vi "Muscolino_v1_KCL.vi"() -> ()   [LabVIEW 2011]
uses:
  <vilib>/DAQmx/read.llb/DAQmx Read (Analog 1D Wfm NChan NSamp).vi
  <vilib>/DAQmx/create/channels.llb/DAQmx Create Channel (AI-Voltage-Basic).vi
  <vilib>/DAQmx/configure/timing.llb/DAQmx Timing (Sample Clock).vi
  <vilib>/DAQmx/configure/task.llb/DAQmx Configure Logging (TDMS).vi
  <vilib>/DAQmx/miscellaneous.llb/DAQmx Fill In Error Info.vi
panel:
  in  "Stimulator":T1={"frequency (Hz)"=1.0, "initial delay (ms)"=100.0, "# Stimuli"=2, "ON-OFF"=TRUE, "pulse dur (ms)"=2.0} {"frequency (Hz)" min=1.0 max=200.0 step=1.0 scale=0.0..100.0}
  in  "Read streamed data":bool
  in  "Play Button":bool
  out "Boolean":bool
  in  "Stop Button":bool
  out "Detector":bool=TRUE
  out "Shutters":bool=TRUE
  in  "Tab Control 3":enum32{"Continuous", "Finite sampling"}(tab)
  in  "ms/point":dbl=1.0
  in  "file path":path=path "C:/Users/Luca/Desktop/BABY"
  in  "ms/point 2":dbl=0.1
  in  "duration (ms)":i32=3000
  in  "Tab Control 2":enum32{"Shutters", "Detector TRG"}(tab)
  in  "Shutter #1":T2={"Duration (ms)"=770.0, "Delay (ms)"=910.0, "# Cycles"=1, "period (ms)"=500.0, "ENABLE"=FALSE}
  in  "Shutter #2":T2={"Duration (ms)"=3.0, "Delay (ms)"=918.0, "# Cycles"=1, "period (ms)"=500.0, "ENABLE"=FALSE}
  in  "TRG detector":T3={"Delay (ms)"=900.0, "Duration (ms)"=1.0, "ENABLE"=TRUE}
  in  "Tab Control":T4(tab)
  out "Waveform Chart 2":waveform(dbl)[](graph)=[{"t0"=timestamp(3645626346.405727 s since 1904-01-01), "dt"=0.001, "Y"=[-0.06398468896060096, -0.06242254708157085, -0.06554683084097776, -0.0664841159698506, -0.06773382947576925, -0.062110118705926365, -0.06273497545726918, -0.06429711733656855, -0.061797690330335706, -0.05929826332754758], "attributes"=variant("NI_ChannelName"=variant(string "Force"), "NI_UnitDescription"=variant(string "Volts"))}, {"t0"=timestamp(3645626346.405727 s since 1904-01-01), "dt"=0.001, "Y"=[10.23122258005124, 10.23122258005124, 10.23122258005124, 10.23122258005124, 10.23122258005124, 10.23122258005124, 10.23122258005124, 10.23122258005124, 10.23122258005124, 10.23122258005124], "attributes"=variant("NI_ChannelName"=variant(string "Motor"), "NI_UnitDescription"=variant(string "Volts"))}, {"t0"=timestamp(3645626346.405727 s since 1904-01-01), "dt"=0.001, "Y"=[0.001985937762198508, 0.01605118530383799, 0.02261496751857621, 0.028241066574480733, 0.03105411610756004, 0.028866188692646493, 0.03636765412387749, 0.02230240646031397, 0.022927528576880348, 0.009174842050874644], "attributes"=variant("NI_ChannelName"=variant(string "Stimulus"), "NI_UnitDescription"=variant(string "Volts"))}]
  out "Waveform Chart":waveform(dbl)[](graph)=[{"t0"=timestamp(3645626346.405727 s since 1904-01-01), "dt"=0.001, "Y"=[-0.06398468896060096, -0.06242254708157085, -0.06554683084097776, -0.0664841159698506, -0.06773382947576925, -0.062110118705926365, -0.06273497545726918, -0.06429711733656855, -0.061797690330335706, -0.05929826332754758], "attributes"=variant("NI_ChannelName"=variant(string "Force"), "NI_UnitDescription"=variant(string "Volts"))}, {"t0"=timestamp(3645626346.405727 s since 1904-01-01), "dt"=0.001, "Y"=[10.23122258005124, 10.23122258005124, 10.23122258005124, 10.23122258005124, 10.23122258005124, 10.23122258005124, 10.23122258005124, 10.23122258005124, 10.23122258005124, 10.23122258005124], "attributes"=variant("NI_ChannelName"=variant(string "Motor"), "NI_UnitDescription"=variant(string "Volts"))}, {"t0"=timestamp(3645626346.405727 s since 1904-01-01), "dt"=0.001, "Y"=[0.001985937762198508, 0.01605118530383799, 0.02261496751857621, 0.028241066574480733, 0.03105411610756004, 0.028866188692646493, 0.03636765412387749, 0.02230240646031397, 0.022927528576880348, 0.009174842050874644], "attributes"=variant("NI_ChannelName"=variant(string "Stimulus"), "NI_UnitDescription"=variant(string "Volts"))}]
  out "Waveform Graph":waveform(dbl)[](graph)=[{"t0"=timestamp(3645626338.6502304 s since 1904-01-01), "dt"=9.999999999999999e-05, "Y"=array[30000 elements], "attributes"=variant("NI_ChannelName"=variant(string "Force"), "NI_UnitDescription"=variant(string "Volts"))}, {"t0"=timestamp(3645626338.6502304 s since 1904-01-01), "dt"=9.999999999999999e-05, "Y"=array[30000 elements], "attributes"=variant("NI_ChannelName"=variant(string "Motor"), "NI_UnitDescription"=variant(string "Volts"))}, {"t0"=timestamp(3645626338.6502304 s since 1904-01-01), "dt"=9.999999999999999e-05, "Y"=array[30000 elements], "attributes"=variant("NI_ChannelName"=variant(string "Stimulus"), "NI_UnitDescription"=variant(string "Volts"))}, {"t0"=timestamp(3645626338.6502304 s since 1904-01-01), "dt"=9.999999999999999e-05, "Y"=array[30000 elements], "attributes"=variant("NI_ChannelName"=variant(string "SH1"), "NI_UnitDescription"=variant(string "Volts"))}, {"t0"=timestamp(3645626338.6502304 s since 1904-01-01), "dt"=9.999999999999999e-05, "Y"=array[30000 elements], "attributes"=variant("NI_ChannelName"=variant(string "SH2"), "NI_UnitDescription"=variant(string "Volts"))}, {"t0"=timestamp(3645626338.6502304 s since 1904-01-01), "dt"=9.999999999999999e-05, "Y"=array[30000 elements], "attributes"=variant("NI_ChannelName"=variant(string "TFG"), "NI_UnitDescription"=variant(string "Volts"))}, {"t0"=timestamp(3645626338.6502304 s since 1904-01-01), "dt"=9.999999999999999e-05, "Y"=array[30000 elements], "attributes"=variant("NI_ChannelName"=variant(string "PIN_DIODE"), "NI_UnitDescription"=variant(string "Volts"))}]
  # "STIMULATOR"
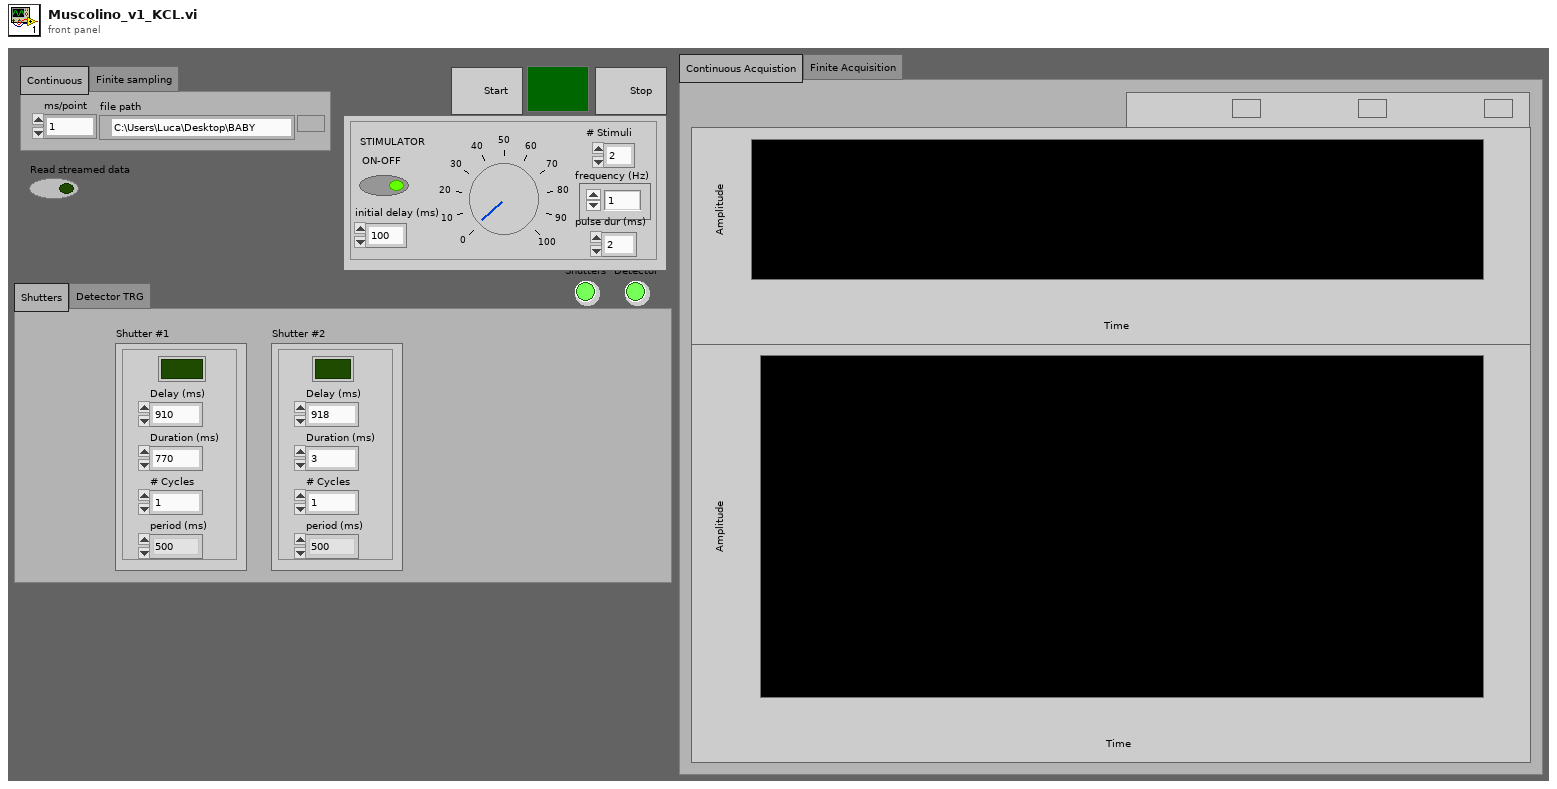
[diagram p1: front panel]
types:
  T1 = cluster{"frequency (Hz)":dbl, "initial delay (ms)":dbl, "# Stimuli":i8, "ON-OFF":bool, "pulse dur (ms)":dbl}
  T2 = cluster{"Duration (ms)":dbl, "Delay (ms)":dbl, "# Cycles":i8, "period (ms)":dbl, "ENABLE":bool}
  T3 = cluster{"Delay (ms)":dbl, "Duration (ms)":dbl, "ENABLE":bool}
  T4 = enum32{"Continuous Acquistion", "Finite Acquisition"}
  T5 = cluster{"data[0]":waveform(dbl), "data[1]":waveform(dbl), "data[2]":waveform(dbl), "data[3]":waveform(dbl), "data[4]":waveform(dbl), "data[5]":waveform(dbl), "data[6]":waveform(dbl), "data[7]":waveform(dbl), "data[8]":waveform(dbl)}
  T6 = cluster{waveform(dbl), waveform(dbl), "data[2]":waveform(dbl)}
  T7 = cluster{"data 2[0]":waveform(dbl), "data 2[1]":waveform(dbl), "data 2[2]":waveform(dbl), "data 2[3]":waveform(dbl), "data 2[4]":waveform(dbl), "data 2[5]":waveform(dbl), "data 2[6]":waveform(dbl), "data 2[7]":waveform(dbl), "data 2[8]":waveform(dbl)}
  T8 = cluster{waveform(dbl), waveform(dbl), "data 2[2]":waveform(dbl), "data 2[3]":waveform(dbl), "data 2[4]":waveform(dbl), "data 2[5]":waveform(dbl), "data 2[6]":waveform(dbl)}
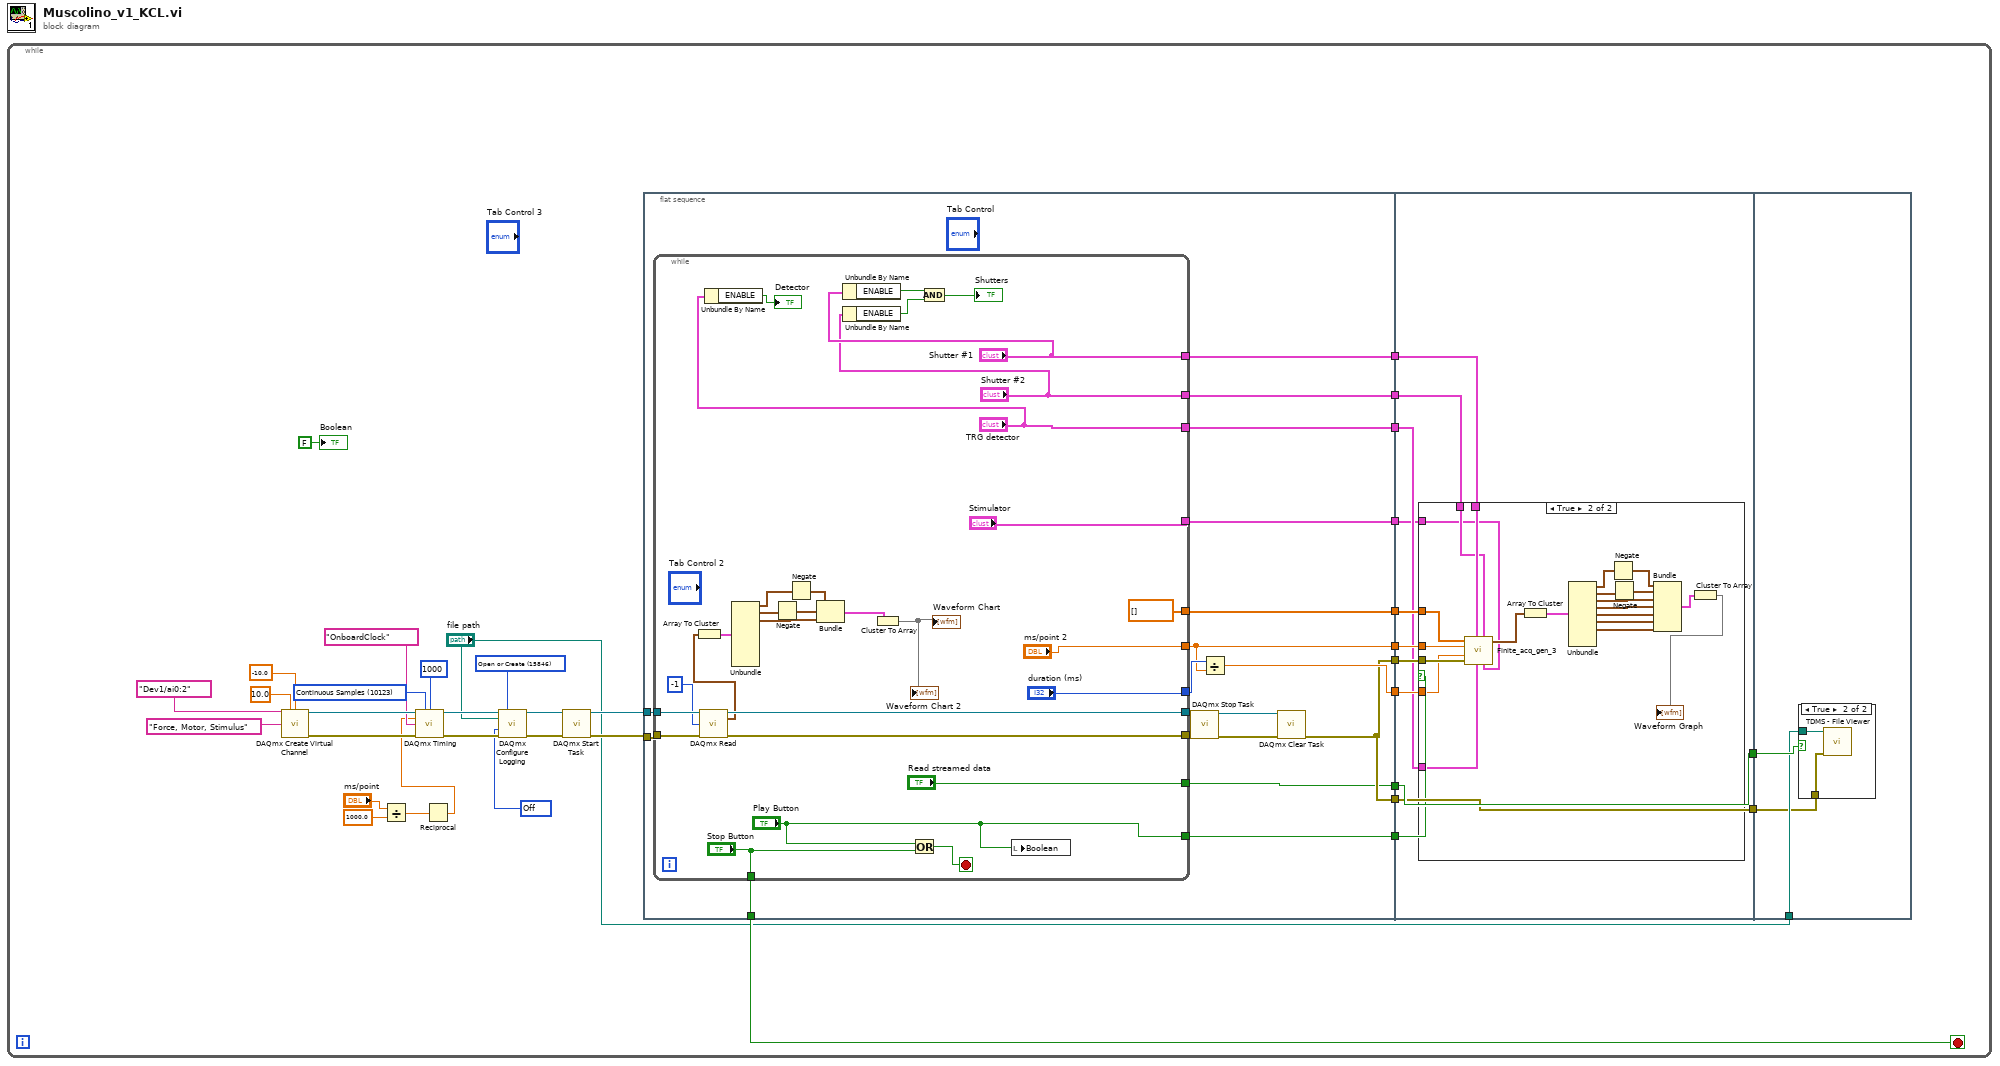
[diagram p0: block diagram]
diagram:
  n1 = while {
    stop <- w23 stop-if-true
    w13 = 15846 items=["Open"=10437, "Open or Create"=15846, "Create or Replace"=15847, "Create"=15848] ("operation")
    w14 = 10231 items=["Off"=10231, "Log"=15844, "Log and Read"=15842] ("logging mode")
    w32 = 10123 items=["Finite Samples"=10178, "Continuous Samples"=10123, "Hardware Timed Single Point"=12522] ("sample mode")
    n2 = call-poly <vilib>:"DAQmx Create Virtual Channel.vi"("maximum value"=10.0, "minimum value"=-10.0, "physical channels"=tag "Dev1/ai0:2", "name to assign"="Force, Motor, Stimulus") -> ("task out"=w33:refnum<k21>, "error out"=w34:errorcluster)  [unwired: 10 in]
    n3 = Divide(x="ms/point", y=1000.0) -> (x/y=w27:dbl)
    n4 = Reciprocal(x=w27) -> (1/x=w25:dbl)
    n5 = call-poly <vilib>:"DAQmx Timing.vi"("task/channels in"=w33, "sample mode"=w32, "samples per channel"=1000, "rate"=w25, "source"=tag "OnboardClock", "error in"=w34) -> ("task out"=w18:refnum<k21>, "error out"=w17:errorcluster)  [unwired: 8 in]
    n6 = call-poly <vilib>:"DAQmx Configure Logging.vi"("task/channels in"=w18, "operation"=w13, "file path"="file path", "logging mode"=w14, "error in"=w17) -> ("task out"=w15:refnum<k21>, "error out"=w16:errorcluster)  [unwired: 9 in]
    n7 = call <vilib>:"DAQmx Start Task.vi"("task/channels in"=w15, "error in"=w16) -> ("task out"=w29:refnum<k21>, "error out"=w24:errorcluster)  [unwired: 12 in]
    n8 = flat-sequence {
      tunnel: w29 -> [w55]
      tunnel: w24 -> [w54]
      tunnel: [w53] -> w23
      tunnel: [w52] -> w22
      tunnel: [w44] -> w21
      tunnel: [w46] -> w20
      tunnel: [w45] -> w19
      tunnel: [w44] -> w12
      tunnel: [w43] -> w11
      tunnel: [w42] -> w7
      tunnel: [w41] -> w4
      tunnel: [w40] -> w3
      tunnel: [w39] -> w2
      tunnel: [w38] -> w1
      tunnel: w22 -> [w95]
      tunnel: w21 -> [w94]
      tunnel: w20 -> [w92]
      tunnel: w19 -> [w93]
      tunnel: w12 -> [w90]
      tunnel: w11 -> [w91]
      tunnel: [w91] -> w10
      tunnel: [w90] -> w9
      tunnel: w7 -> [w89]
      tunnel: w4 -> [w88]
      tunnel: w3 -> [w87]
      tunnel: w2 -> [w86]
      tunnel: w1 -> [w85]
      tunnel: w10 -> [w119]
      tunnel: w9 -> [w117]
      tunnel: "file path" -> [w118]
      frame #0 {
        n9 = while {
          tunnel: w55 -> [w84]
          tunnel: [w83] -> w49
          tunnel: [w82] -> w51
          tunnel: w54 -> [w80]
          tunnel: ["Stop Button"] -> w53
          tunnel: [dbl[] [] ("Anolog. array")] -> w52
          tunnel: ["ms/point 2"] -> w46
          tunnel: ["duration (ms)"] -> w47
          tunnel: ["Read streamed data"] -> w43
          tunnel: ["Play Button"] -> w42
          tunnel: ["Shutter #1"] -> w41
          tunnel: ["Shutter #2"] -> w40
          tunnel: ["TRG detector"] -> w39
          tunnel: ["Stimulator"] -> w38
          stop <- w79 stop-if-true
          n10 = call-poly <vilib>:"DAQmx Read.vi"("task/channels in"=w84, "number of samples per channel"=-1, "error in"=w80) -> ("task out"=w82:refnum<k21>, "data"=w75:waveform(dbl)[], "error out"=w83:errorcluster)  [unwired: 10 in]
          n11 = Array To Cluster(array=w75) -> (cluster=w74:T5)
          n12 = Unbundle By Name("TRG detector") -> ("ENABLE"=→"Detector":bool)
          n13 = Unbundle(w74) -> ("data[0]"=w59:waveform(dbl), "data[1]"=w71:waveform(dbl), "data[2]"=w72:waveform(dbl))  [unwired: 6 out]
          n14 = Negate(x=w71) -> (-x=w70:waveform(dbl))
          n15 = Negate(x=w59) -> (-x=w58:waveform(dbl))
          n16 = Bundle(w58, w70, "data[2]"=w72) -> (w73:T6)  [unwired: 1 in]
          n17 = Unbundle By Name("Shutter #1") -> ("ENABLE"=w64:bool)
          n18 = Unbundle By Name("Shutter #2") -> ("ENABLE"=w62:bool)
          n19 = Cluster To Array(cluster=w73) -> (array=→"Waveform Chart" →"Waveform Chart 2":waveform(dbl)[])
          n20 = Or(x="Play Button", y="Stop Button") -> (x .or. y?=w79:bool)
          n21 = And(x=w64, y=w62) -> (x .and. y?=→"Shutters":bool)
          n22 = local write "Boolean"("Play Button") -> ()
        }
        n23 = call <vilib>:"DAQmx Stop Task.vi"("task/channels in"=w51, "error in"=w49) -> ("task out"=w50:refnum<k21>, "error out"=w48:errorcluster)  [unwired: 12 in]
        n24 = Divide(x=w47, y=w46) -> (x/y=w45:dbl)
        n25 = call <vilib>:"DAQmx Clear Task.vi"("task in"=w50, "error in"=w48) -> ("error out"=w44:errorcluster)  [unwired: 13 in]
      }
      frame #1 {
        n26 = case shown="True" w89 {
          tunnel: w95 -> [_ w116]
          tunnel: w94 -> [_ w115]
          tunnel: w93 -> [_ w114]
          tunnel: w92 -> [_ w113]
          tunnel: w88 -> [_ w104]
          tunnel: w87 -> [_ w103]
          tunnel: w86 -> [_ w102]
          tunnel: w85 -> [_ w96]
          frame False {
          }
          frame True {
            n27 = call "Finite_acq_gen_3.vi"("Stimulator"=w96, "Shutter #2"=w103, "TRG detector"=w102, "Shutter #1"=w104, "error in"=w115, "samples per channel"=w114, "ms/point"=w113, "data"=w116) -> ("data 2"=w107:waveform(dbl)[])  [unwired: 3 in]
            n28 = Array To Cluster(array=w107) -> (cluster=w112:T7)
            n29 = Unbundle(w112) -> ("data 2[0]"=w98:waveform(dbl), "data 2[1]"=w109:waveform(dbl), "data 2[2]"=w111:waveform(dbl), "data 2[3]"=w110:waveform(dbl), "data 2[4]"=w101:waveform(dbl), "data 2[5]"=w100:waveform(dbl), "data 2[6]"=w99:waveform(dbl))  [unwired: 2 out]
            n30 = Negate(x=w98) -> (-x=w97:waveform(dbl))
            n31 = Negate(x=w109) -> (-x=w108:waveform(dbl))
            n32 = Bundle(w97, w108, "data 2[2]"=w111, "data 2[3]"=w110, "data 2[4]"=w101, "data 2[5]"=w100, "data 2[6]"=w99) -> (w106:T8)  [unwired: 1 in]
            n33 = Cluster To Array(cluster=w106) -> (array=→"Waveform Graph":waveform(dbl)[])
          }
        }
      }
      frame #2 {
        n34 = case shown="True" w119 {
          tunnel: w117 -> [_ w121]
          tunnel: w118 -> [_ w120]
          frame False {
          }
          frame True {
            n35 = call <vilib>:"TDMS - File Viewer.vi"("error in (no error)"=w121, "file path"=w120) -> ()  [unwired: 4 in, 2 out]
          }
        }
      }
    }
    "Boolean" <- FALSE ("Boolean")
  }
